vi "get_config_cluster.vi"(8 "error in (no error)":errorcluster, 11 "SignalReaderMT120810DAQmxOversampling in":refnum<class "SignalReaderMT120810DAQmxOversampling.lvclass">) -> (0 "error out":errorcluster, 2 "config cluster (variant)":variant, 3 "SignalReaderMT120810DAQmxOversampling out":refnum<class "SignalReaderMT120810DAQmxOversampling.lvclass">)   [LabVIEW 2010, in "SignalReaderMT120810DAQmxOversampling.lvclass"]
uses:
  SignalReaderMT120810DAQmxOversampling.lvclass
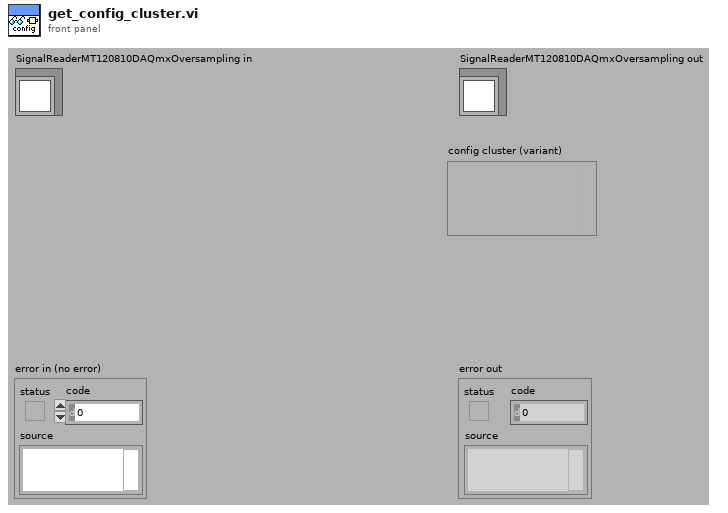
[diagram p1: front panel]
types:
  T1 = typedef "SignalReaderMT120810DAQmxOversampling.lvclass/ChannelDefinition.ctl" = cluster{"physical Channel":string, "max_input_value":dbl, "min_input_value":dbl, "ground_reference":i32, "translation_factor":dbl, "translation_offset":dbl}
  T2 = cluster{"analog input channels":T1[], "clock source":string, "time-out":dbl[unit], "maximum sampling rate":dbl[unit], "buffer size":i32}
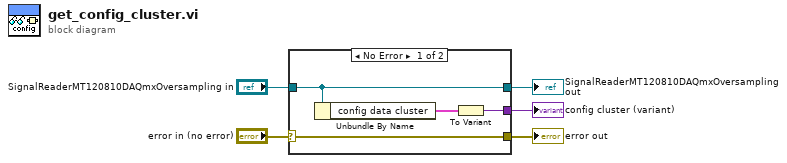
[diagram p0: block diagram]
diagram:
  n1 = case shown="No Error" "error in (no error)" {
    selector: "error in (no error)" -> [w9 w11]
    tunnel: "SignalReaderMT120810DAQmxOversampling in" -> [w8 w10]
    tunnel: [w8 w10] -> w3
    tunnel: [w9 w11] -> w2
    tunnel: [w6 _] -> w1
    frame No Error {
      n2 = Unbundle By Name(w8) -> ("config data cluster"=w7:T2)
      n3 = To Variant(anything=w7) -> (Variant=w6:variant)
    }
    frame Error {
    }
  }
  "error out" <- w2
  "SignalReaderMT120810DAQmxOversampling out" <- w3
  "config cluster (variant)" <- w1
